vi "Set Scale Name.vi"(8 "error in (no error)":errorcluster, 9 "references":T1, 10 "name":string, 11 "index":i32) -> (0 "error out":errorcluster)   [LabVIEW 2013, in "Scaling configuration.lvclass"]
uses:
  Scaling configuration.lvclass
  <vilib>/NI/DCAF Table API/Table Manager/object ref.ctl
  <vilib>/NI/Tag Bus Data Framework/Configuration Editor/Classes/Engine Parent/Engine Parent Editor Node.lvclass
  <vilib>/NI/Tag Bus Data Framework/Configuration Editor/Classes/Module editor node/module editor node.lvclass
  Scaling configuration.lvclass/Scaling configuration.ctl
  <vilib>/NI/DCAF Table API/Table Manager/Table Manager.lvclass
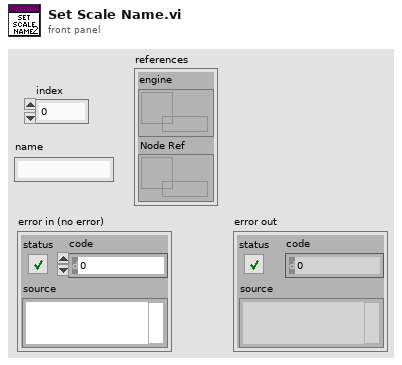
[diagram p1: front panel]
types:
  T1 = typedef "Table Manager.lvlib/Table Manager.lvclass/object ref.ctl" = cluster{"engine":refnum<data-value>, "Node Ref":refnum<data-value>}
  T2 = typedef "Scaling configuration.lvclass/scale data types.ctl" = enum16{"Double", "Single", "I64", "I32", "I16", "I8", "U64", "U32", "U16", "U8"}
  T3 = cluster{"mappings":cluster{"input channel":refnum<class "TBM channel.lvclass">, "output channel":refnum<class "TBM channel.lvclass">, "input data type":T2, "output data type":T2}[], "name":string}[]
  T4 = cluster{"mappings":cluster{"input channel":refnum<class "TBM channel.lvclass">, "output channel":refnum<class "TBM channel.lvclass">, "input data type":T2, "output data type":T2}[], "name":string}
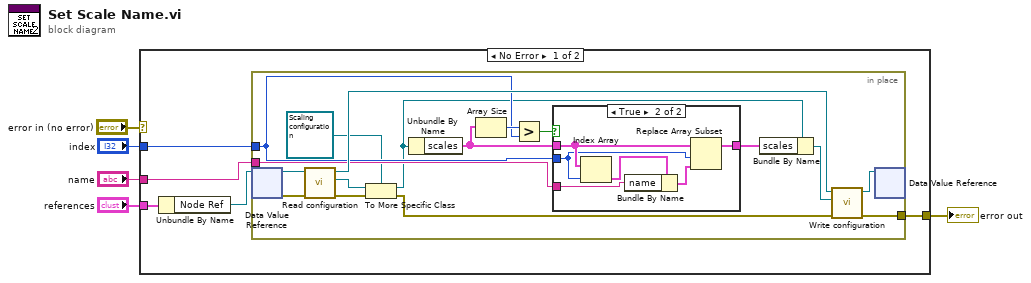
[diagram p0: block diagram]
diagram:
  n1 = case shown="No Error" "error in (no error)" {
    selector: "error in (no error)" -> [_ w35]
    tunnel: [w10 w35] -> w3
    tunnel: "index" -> [w8 _]
    tunnel: "references" -> [w7 _]
    tunnel: "name" -> [w6 _]
    frame No Error {
      n2 = Unbundle By Name(w7) -> ("Node Ref"=w9:refnum<data-value>)
      n3 = in-place {
        in-place-border: [w23] -> w10
        in-place-border: w8 -> [w17]
        in-place-border: w6 -> [w16]
        n4 = in-place-dvr #1(w9) -> (w26:refnum<class "module editor node.lvclass">, w22:errorcluster)
        n5 = call-dynamic "Read configuration.vi"("error in"=w22, "NISE_CEF_serializable node in"=w26) -> ("error out"=w21:errorcluster, "configuration"=w25:refnum<class "NISE_CEF_serializable configuration.lvclass">, "NISE_CEF_serializable node out"=w27:refnum<class "module editor node.lvclass">)  [unwired: 7 in]
        n6 = To More Specific Class(target class=refnum<class "Scaling configuration.lvclass"> refnum ("Scaling configuration"), reference=w25, error in=w21) -> (specific class reference=w11:refnum<class "Scaling configuration.lvclass">, error out=w13:errorcluster)
        n7 = Unbundle By Name(w11) -> ("scales"=w18:T3)
        n8 = Array Size(array=w18) -> (size(s)=w20:i32)
        n9 = Greater?(x=w20, y=w17) -> (0:w19:bool)
        n10 = case shown="True" w19 {
          tunnel: w18 -> [w28 w33]
          tunnel: w17 -> [_ w32]
          tunnel: w16 -> [_ w34]
          tunnel: [w28 w30] -> w15
          frame False {
          }
          frame True {
            n11 = Index Array(array=w33, index=w32) -> (element=w31:T4)
            n12 = Bundle By Name(cluster=w31, "name"=w34) -> (w29:T4)
            n13 = Replace Array Subset(array=w33, new element=w29, index=w32) -> (w30:T3)
          }
        }
        n14 = Bundle By Name(cluster=w11, "scales"=w15) -> (w14:refnum<class "Scaling configuration.lvclass">)
        n15 = call-dynamic "Write configuration.vi"("error in"=w13, "configuration"=w14, "NISE_CEF_serializable node in"=w27) -> ("error out"=w23:errorcluster, "NISE_CEF_serializable node out"=w24:refnum<class "module editor node.lvclass">)  [unwired: 7 in]
        n16 = in-place-dvr #1(w24) -> ()  [unwired: 2 out]
      }
    }
    frame Error {
    }
  }
  "error out" <- w3
